vi "RehomeLift.vi"(11 "array":bool[](array[boolean])) -> ()   [LabVIEW 2014]
uses:
  <vilib>/Rock Robotics/WPI/CAN/TalonSRX/WPI_CANTalonSRX_APIControlMode.ctl
  <vilib>/Rock Robotics/WPI/CAN/TalonSRX/WPI_CANTalonSRX_APIFeedbackSelect.ctl
panel:
  in  "Lift PID Gains":T1={"proportional gain (Kc)"=120.0, "integral time (Ti, min)"=0.0, "derivative time (Td, min)"=85.0}
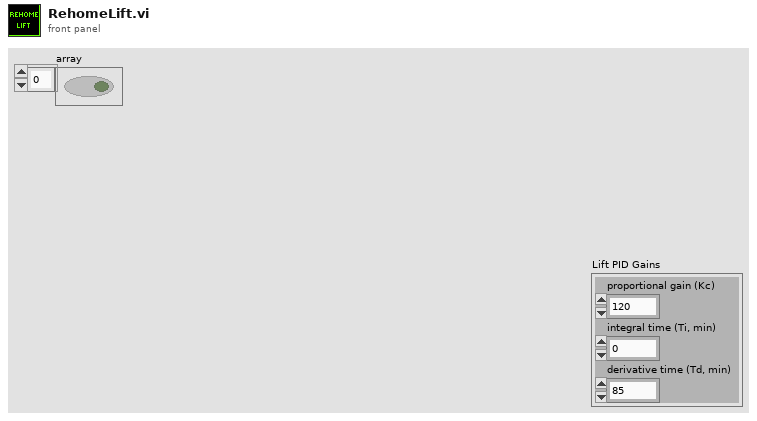
[diagram p1: front panel]
types:
  T1 = cluster{"proportional gain (Kc)":dbl, "integral time (Ti, min)":dbl, "derivative time (Td, min)":dbl}
  T2 = typedef "WPI_CANTalonSRX_APIFeedbackSelect.ctl" = enum16{"Digital Quadrature Encoder", "Analog Potentiometer", "Analog Encoder"}
  T3 = typedef "WPI_CANTalonSRX_APIControlMode.ctl" = enum8{"Percent VBus", "Speed", "Position", "Slave", "Unchanged / Invalid"}
  T4 = typedef "WPI_MotorControlDeviceRef.ctl" = cluster{"DeviceStatus":errorcluster, "Type":T5, "PWM":cluster{"Controller":T6, "PWM Channel":T7, "DeadBand":T8}, "CAN":cluster{"Device Number":u8, "Control Mode":T9, "Semaphore":T10, "Max Vout":dbl, "TalonSRX Control Mode":T3}, "Invert":bool, "TransformRef":T11, "InvTransformRef":T11}
  T5 = typedef "WPI_MotorControlType.ctl" = enum16{"PWM", "CAN", "CANTalonSRX"}
  T6 = typedef "FPGA_TypedefDigitalModule.ctl" = enum16{"Controller 1"}
  T7 = typedef "FPGA_DIOPWMChannel.ctl" = enum8{"PWM 0", "PWM 1", "PWM 2", "PWM 3", "PWM 4", "PWM 5", "PWM 6", "PWM 7", "PWM 8", "PWM 9", "PWM MXP 0", "PWM MXP 1", "PWM MXP 2", "PWM MXP 3", "PWM MXP 4", "PWM MXP 5", "PWM MXP 6", "PWM MXP 7", "PWM MXP 8", "PWM MXP 9", "Invalid"}
  T8 = typedef "WPI_PWMDeadband.ctl" = cluster{"Name":string, "maxPositivePwm":i32, "minPositivePwm":i32, "centerPwm":i32, "maxNegativePwm":i32, "minNegativePwm":i32, "angularRange":u16}
  T9 = typedef "WPI_CANJaguar_ControlMode.ctl" = enum8{"Percent VBus", "Current", "Speed", "Position", "Voltage"}
  T10 = typedef "Semaphore RefNum" = refnum<k1>
  T11 = typedef "WPI_PWMTransform_ConPane.ctl" = refnum<vi>
  T12 = typedef "WPI_CANTalonSRX_GlobalStatus.ctl" = cluster{"Applied Throttle":dbl, "Module Enabled":bool, "CAN Error":errorcluster, "Closed Loop Error":dbl, "Forward Limit Switch Closed":bool, "Reverse Limit Switch Closed":bool, "Sensor Position":dbl, "Sensor Velocity":dbl, "Current":dbl, "Sticky Fault - Over Temp":bool, "Sticky Fault - Under Voltage":bool, "Sticky Fault - Forward Limit":bool, "Sticky Fault - Reverse Limit":bool, "Sticky Fault - Forward Soft Limit":bool, "Sticky Fault - Reverse Soft Limit":bool, "Brake is Enabled":bool, "Encoder Position":dbl, "Encoder Velocity":dbl, "Encoder Index Count":dbl, "Encoder A Pin State":bool, "Encoder B Pin State":bool, "Encoder Index Pin State":bool, "Analog In":dbl, "Analog In Velocity":dbl, "Temperature (C)":dbl, "Battery Voltage":dbl}
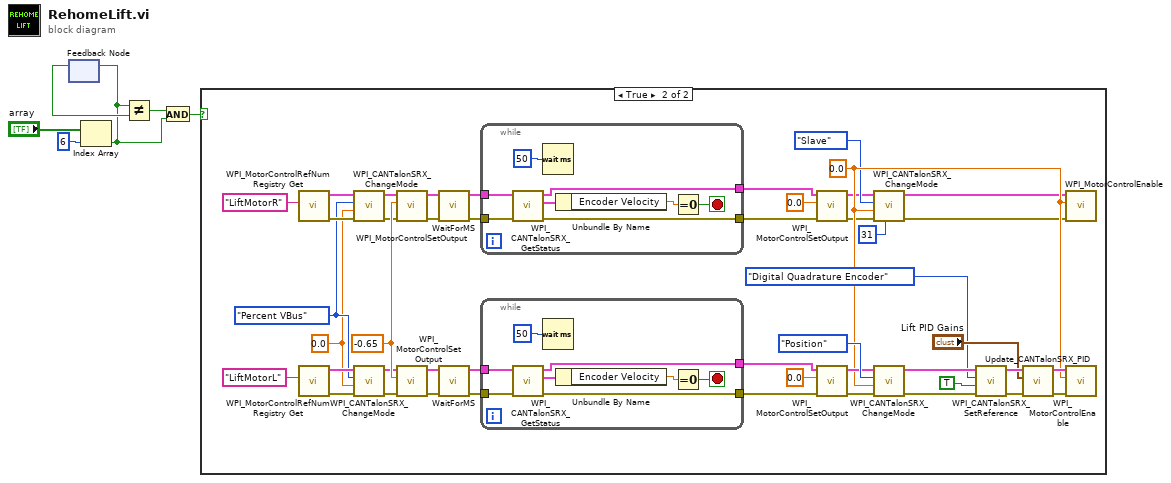
[diagram p0: block diagram]
diagram:
  n1 = feedback #1() -> (w6:bool)  [unwired: 1 in]
  n2 = Index Array(array="array", index=6) -> (element=w2:bool)
  n3 = feedback-in #1(w2) -> ()
  n4 = Not Equal?(x=w2, y=w6) -> (x != y?=w5:bool)
  n5 = And(x=w5, y=w2) -> (x .and. y?=w4:bool)
  n6 = case shown="True" w4 {
    frame False {
    }
    frame True {
      w14 = 0.0 ("Output")
      w15 = WPI_CANTalonSRX_APIControlMode."Percent VBus" ("Control Mode")
      w36 = 0.0 ("Output")
      w38 = -0.65 ("Output")
      n7 = call <vilib>:"WPI_MotorControlRefNum Registry Get.vi"("refnum name"="LiftMotorR") -> ("error out"=w16:errorcluster, "MotorControlDevRef"=w17:T4)  [unwired: 9 in]
      n8 = call <vilib>:"WPI_MotorControlRefNum Registry Get.vi"("refnum name"="LiftMotorL") -> ("error out"=w18:errorcluster, "MotorControlDevRef"=w19:T4)  [unwired: 9 in]
      n9 = call <vilib>:"WPI_CANTalonSRX_ChangeMode.vi"("error in (no error)"=w16, "Output"=w14, "Control Mode"=w15, "CAN Talon SRX Ref"=w17) -> ("error out"=w10:errorcluster, "CAN Talon SRX Ref Out"=w11:T4)  [unwired: 6 in]
      n10 = call <vilib>:"WPI_CANTalonSRX_ChangeMode.vi"("error in (no error)"=w18, "Output"=w14, "Control Mode"=w15, "CAN Talon SRX Ref"=w19) -> ("error out"=w12:errorcluster, "CAN Talon SRX Ref Out"=w13:T4)  [unwired: 6 in]
      n11 = call <vilib>:"WPI_MotorControlSetOutput.vi"("error in (no error)"=w10, "Output"=w38, "MotorControlDevRef"=w11) -> ("error out"=w23:errorcluster, "MotorControlDevRef"=w24:T4)  [unwired: 6 in, 1 out]
      n12 = call <vilib>:"WPI_MotorControlSetOutput.vi"("error in (no error)"=w12, "Output"=w38, "MotorControlDevRef"=w13) -> ("error out"=w34:errorcluster, "MotorControlDevRef"=w35:T4)  [unwired: 6 in, 1 out]
      n13 = call "WaitForMS.vi"("error in"=w23, "MotorControlDevRef"=w24) -> ("error out"=w21:errorcluster, "MotorControlDevRef 2"=w22:T4)  [unwired: 8 in]
      n14 = call "WaitForMS.vi"("error in"=w34, "MotorControlDevRef"=w35) -> ("error out"=w33:errorcluster, "MotorControlDevRef 2"=w32:T4)  [unwired: 8 in]
      n15 = while {
        tunnel: w22 -> [w59]
        tunnel: w21 -> [w58]
        tunnel: [w55] -> w26
        tunnel: [w54] -> w25
        stop <- w53 stop-if-true
        n16 = call <vilib>:"WPI_CANTalonSRX_GetStatus.vi"("error in (no error)"=w58, "CAN Talon SRX Ref"=w59) -> ("error out"=w54:errorcluster, "Talon SRX Status"=w57:T12, "CAN Talon SRX Ref Out"=w55:T4)  [unwired: 7 in]
        n17 = Wait (ms)(milliseconds to wait=u32 50) -> ()  [unwired: 1 out]
        n18 = Unbundle By Name(w57) -> ("Encoder Velocity"=w56:dbl)
        n19 = Equal To 0?(x=w56) -> (x = 0?=w53:bool)
      }
      n20 = while {
        tunnel: w32 -> [w67]
        tunnel: w33 -> [w66]
        tunnel: [w64] -> w40
        tunnel: [w63] -> w39
        stop <- w61 stop-if-true
        n21 = call <vilib>:"WPI_CANTalonSRX_GetStatus.vi"("error in (no error)"=w66, "CAN Talon SRX Ref"=w67) -> ("error out"=w63:errorcluster, "Talon SRX Status"=w65:T12, "CAN Talon SRX Ref Out"=w64:T4)  [unwired: 7 in]
        n22 = Wait (ms)(milliseconds to wait=u32 50) -> ()  [unwired: 1 out]
        n23 = Unbundle By Name(w65) -> ("Encoder Velocity"=w62:dbl)
        n24 = Equal To 0?(x=w62) -> (x = 0?=w61:bool)
      }
      n25 = call <vilib>:"WPI_MotorControlSetOutput.vi"("error in (no error)"=w25, "Output"=0.0, "MotorControlDevRef"=w26) -> ("error out"=w27:errorcluster, "MotorControlDevRef"=w28:T4)  [unwired: 6 in, 1 out]
      n26 = call <vilib>:"WPI_MotorControlSetOutput.vi"("error in (no error)"=w39, "Output"=0.0, "MotorControlDevRef"=w40) -> ("error out"=w48:errorcluster, "MotorControlDevRef"=w49:T4)  [unwired: 6 in, 1 out]
      n27 = call <vilib>:"WPI_CANTalonSRX_ChangeMode.vi"("Master Device Number"=u8 31, "error in (no error)"=w27, "Output"=w36, "Control Mode"=WPI_CANTalonSRX_APIControlMode."Slave", "CAN Talon SRX Ref"=w28) -> ("error out"=w7:errorcluster, "CAN Talon SRX Ref Out"=w8:T4)  [unwired: 5 in]
      n28 = call <vilib>:"WPI_CANTalonSRX_ChangeMode.vi"("error in (no error)"=w48, "Output"=w36, "Control Mode"=WPI_CANTalonSRX_APIControlMode."Position", "CAN Talon SRX Ref"=w49) -> ("error out"=w45:errorcluster, "CAN Talon SRX Ref Out"=w44:T4)  [unwired: 6 in]
      n29 = call <vilib>:"WPI_CANTalonSRX_SetReference.vi"("error in (no error)"=w45, "Reverse Feedback Sensor"=TRUE, "Feedback Reference"=WPI_CANTalonSRX_APIFeedbackSelect."Digital Quadrature Encoder", "CAN Talon SRX Ref"=w44) -> ("error out"=w42:errorcluster, "CAN Talon SRX Ref Out"=w43:T4)  [unwired: 6 in]
      n30 = call "Update_CANTalonSRX_PID.vi"("error in (no error)"=w42, "PID Gains"="Lift PID Gains", "CAN Talon SRX Ref"=w43) -> ("error out"=w46:errorcluster, "CAN Talon SRX Ref Out"=w47:T4)  [unwired: 7 in]
      n31 = call <vilib>:"WPI_MotorControlEnable.vi"("error in (no error)"=w7, "Encoder Initial Position"=w36, "CAN Jaguar Ref"=w8) -> ()  [unwired: 7 in, 2 out]
      n32 = call <vilib>:"WPI_MotorControlEnable.vi"("error in (no error)"=w46, "Encoder Initial Position"=w36, "CAN Jaguar Ref"=w47) -> ()  [unwired: 7 in, 2 out]
    }
  }
